vi "Transform to Task.vi"(9 "Line":i8, 10 "Port":i8, 11 "DAQmx Device Name":tag) -> (3 "Classic DAQmx Physical Channel":tag)   [LabVIEW 2016, in "Generic Data Acquisition.lvlib" / "National Instrument USB-6501.lvlib" / "National Instrument USB-6501.lvclass"]
uses:
  National Instrument USB-6501.lvclass
  <resource>/objmgr/daqmx.rc
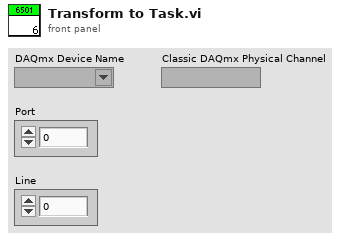
[diagram p1: front panel]
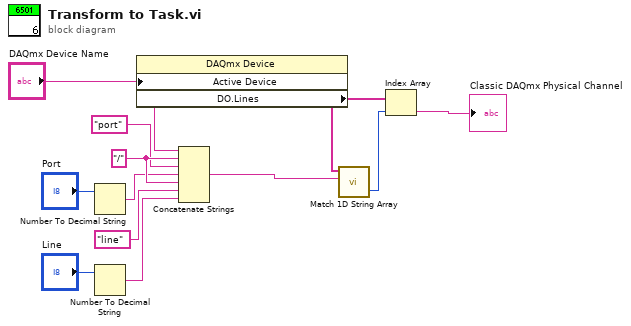
[diagram p0: block diagram]
diagram:
  w3 = "/" ("string")
  n1 = Number To Decimal String(number="Port") -> (decimal integer string=w1:string)  [unwired: 1 in]
  n2 = Number To Decimal String(number="Line") -> (decimal integer string=w5:string)  [unwired: 1 in]
  n3 = property class="DAQmx Device"("Active Device"="DAQmx Device Name") -> ("DO.Lines"=w10:tag[])  [unwired: 2 in, 2 out]
  n4 = Concatenate Strings("DAQmx Device Name", w3, "port" ("string"), w1, w3, "line" ("string"), w5) -> (w9:string)
  n5 = call <vilib>:"Match 1D String Array.vi"("Pattern"=w9, "Strings"=w10) -> ("index of element"=w11:i32)  [unwired: 2 in, 1 out]
  n6 = Index Array(array=w10, index=w11) -> (element=→"Classic DAQmx Physical Channel":tag)
